vi "TelemetryMemoryUpdate.vi"   [LabVIEW 2018]
uses:
  <vilib>/rvi/Emulation/niFpgaGetClockAttributes.vi
  <vilib>/rvi/Emulation/niFpgaSctlEmulationGetInTimedLoop.vi
  <vilib>/rvi/Emulation/niFpgaEmulationReportErrorSimple.vi
  <vilib>/rvi/Emulation/niFpgaEmulationIsFPGAContextNoSignature.vi
  <vilib>/rvi/errors/niFpgaSetErrorForExecOnDevCompSimple.vi
  <vilib>/rvi/eio/common/nirviEmuReportErrorAndStop.vi
  <vilib>/rvi/DataTransferAndStorage/Container/Common/niFpgaContainerGetUniqueNameForEmu.vi
  <vilib>/rvi/FIFO/Fifo_Resource/nirvififoEmulationSetSize.vi
  <vilib>/rvi/FIFO/Fifo_Resource/nirviFifoEmulationQueueMgr.vi
  <instcachedir>/0/nirviFifoEmulationQueueMgr_E5CAEC123FF24DC58D834DCA3CDAA9B5.lvgen/nirviFifoEmulationQueueMgr_E5CAEC123FF24DC58D834DCA3CDAA9B5_022.vi
  <vilib>/Utility/error.llb/Clear Errors.vi
  <vilib>/rvi/FIFO/Fifo_Resource/nirvififoEmulationCreateLock.vi
  <vilib>/rvi/Emulation/niFpgaProcessEmulError.vi
  <vilib>/rvi/FIFO/Fifo_Resource/nirvififoEmulationObtainLock.vi
  <vilib>/rvi/FIFO/Fifo_Resource/nirvififoEmulationReleaseLock.vi
  <vilib>/rvi/occurrence/nirviWaitOnOccurrenceBase.vi
  <vilib>/rvi/errors/nirviReportUnexpectedCaseInternalError.vi
  <vilib>/rvi/errors/nirviReportUnexpectedCaseInternalError (U32).vi
  <vilib>/rvi/Emulation/niFpgaCriticalErrorInLSC.vi
  <vilib>/rvi/DataTransferAndStorage/Container/XNode/niFpgaContainer.xnode
  <vilib>/rvi/FIFO/Fifo_Resource/nirvififoEmulationRead.vi
types:
  T1 = cluster{"DataType":enum8{"U8", "U16", "U32", "U64", "I8", "I16", "I32", "I64", "SGL"}, "Mode":enum8{"=", "+", "-", "|"}, "Field":enum16{"None", "AnalogInputSampleCount", "AnalogInputSampleTimestamp", "AnalogInputRaw1", "AnalogInputRaw2", "AnalogInputRaw3", "AnalogInputRaw4", "AnalogInputRaw5", "AnalogInputRaw6", "AnalogInputRaw7", "AnalogInputRaw8", "AnalogInputRaw9", "AnalogInputRaw10", "AnalogInputRaw11", "AnalogInputRaw12", "AnalogInputRaw13", "AnalogInputRaw14", "AnalogInputRaw15", "AnalogInputRaw16", "DigitalInputSampleCount", "DigitalInputSampleTimestamp", "DigitalInputStates", "ThermocoupleSampleCount", "ThermocoupleSampleTimestamp", "ThermocoupleRaw1", "ThermocoupleRaw2", "ThermocoupleRaw3", "ThermocoupleRaw4", "ThermocoupleRaw5", "ThermocoupleRaw6", "ThermocoupleRaw7", "ThermocoupleRaw8", "ThermocoupleRaw9", "ThermocoupleRaw10", "ThermocoupleRaw11", "ThermocoupleRaw12", "ThermocoupleRaw13", "ThermocoupleRaw14", "ThermocoupleRaw15", "ThermocoupleRaw16", "WindSensorTxBytes", "WindSensorTxFrames", "WindSensorRxBytes", "WindSensorRxFrames", "WindSensorErrorTimestamp", "WindSensorErrorCode", "WindSensorSampleTimestamp", "WindSensorXRaw", "WindSensorYRaw", "WindSensorZRaw", "WindSensorSonicTempRaw", "WindSensorDiagWord", "WindSensorRecordCount", "FlowSensorTxBytes", "FlowSensorTxFrames", "FlowSensorRxBytes", "FlowSensorRxFrames", "FlowSensorErrorTimestamp", "FlowSensorErrorCode", "FlowSensorSampleTimestamp", "FlowSensorSignalStrength", "FlowSensorFlowRate", "FlowSensorNetTotalizer", "FlowSensorPositiveTotalizer", "FlowSensorNegativeTotalizer", "FlowSensorTemperature1", "FlowSensorTemperature2", "VFDTxBytes", "VFDTxFrames", "VFDRxBytes", "VFDRxFrames", "VFDErrorTimestamp", "VFDErrorCode", "VFDSampleTimestamp", "VFDVelocityBits", "VFDDiagnosticCode", "VFDFrequencyCommand", "VFDOutputFrequency", "VFDOutputCurrent", "VFDDCBusVoltage", "VFDOutputVoltage"}, "Data":u64}
  T2 = enum8{"U8", "U16", "U32", "U64", "I8", "I16", "I32", "I64", "SGL"}
  T3 = enum16{"None", "AnalogInputSampleCount", "AnalogInputSampleTimestamp", "AnalogInputRaw1", "AnalogInputRaw2", "AnalogInputRaw3", "AnalogInputRaw4", "AnalogInputRaw5", "AnalogInputRaw6", "AnalogInputRaw7", "AnalogInputRaw8", "AnalogInputRaw9", "AnalogInputRaw10", "AnalogInputRaw11", "AnalogInputRaw12", "AnalogInputRaw13", "AnalogInputRaw14", "AnalogInputRaw15", "AnalogInputRaw16", "DigitalInputSampleCount", "DigitalInputSampleTimestamp", "DigitalInputStates", "ThermocoupleSampleCount", "ThermocoupleSampleTimestamp", "ThermocoupleRaw1", "ThermocoupleRaw2", "ThermocoupleRaw3", "ThermocoupleRaw4", "ThermocoupleRaw5", "ThermocoupleRaw6", "ThermocoupleRaw7", "ThermocoupleRaw8", "ThermocoupleRaw9", "ThermocoupleRaw10", "ThermocoupleRaw11", "ThermocoupleRaw12", "ThermocoupleRaw13", "ThermocoupleRaw14", "ThermocoupleRaw15", "ThermocoupleRaw16", "WindSensorTxBytes", "WindSensorTxFrames", "WindSensorRxBytes", "WindSensorRxFrames", "WindSensorErrorTimestamp", "WindSensorErrorCode", "WindSensorSampleTimestamp", "WindSensorXRaw", "WindSensorYRaw", "WindSensorZRaw", "WindSensorSonicTempRaw", "WindSensorDiagWord", "WindSensorRecordCount", "FlowSensorTxBytes", "FlowSensorTxFrames", "FlowSensorRxBytes", "FlowSensorRxFrames", "FlowSensorErrorTimestamp", "FlowSensorErrorCode", "FlowSensorSampleTimestamp", "FlowSensorSignalStrength", "FlowSensorFlowRate", "FlowSensorNetTotalizer", "FlowSensorPositiveTotalizer", "FlowSensorNegativeTotalizer", "FlowSensorTemperature1", "FlowSensorTemperature2", "VFDTxBytes", "VFDTxFrames", "VFDRxBytes", "VFDRxFrames", "VFDErrorTimestamp", "VFDErrorCode", "VFDSampleTimestamp", "VFDVelocityBits", "VFDDiagnosticCode", "VFDFrequencyCommand", "VFDOutputFrequency", "VFDOutputCurrent", "VFDDCBusVoltage", "VFDOutputVoltage"}
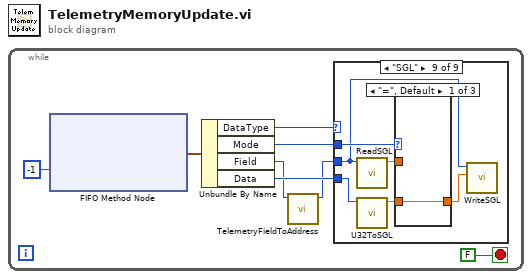
[diagram p0: block diagram]
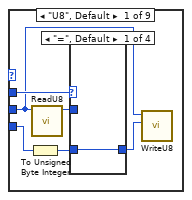
[diagram p2: hidden frame]
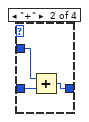
[diagram p3: hidden frame]
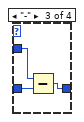
[diagram p4: hidden frame]
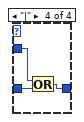
[diagram p5: hidden frame]
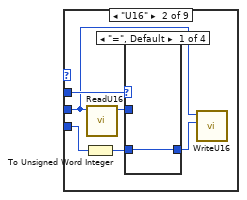
[diagram p6: hidden frame]
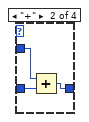
[diagram p7: hidden frame]
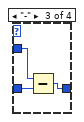
[diagram p8: hidden frame]
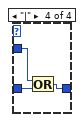
[diagram p9: hidden frame]
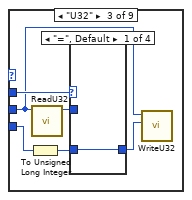
[diagram p10: hidden frame]
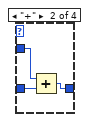
[diagram p11: hidden frame]
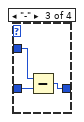
[diagram p12: hidden frame]
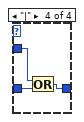
[diagram p13: hidden frame]
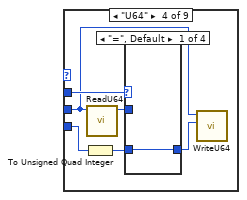
[diagram p14: hidden frame]
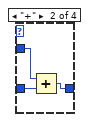
[diagram p15: hidden frame]
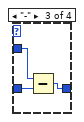
[diagram p16: hidden frame]
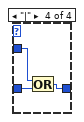
[diagram p17: hidden frame]
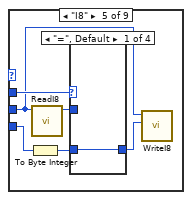
[diagram p18: hidden frame]
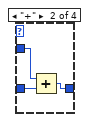
[diagram p19: hidden frame]
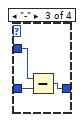
[diagram p20: hidden frame]
diagram:
  n1 = while {
    stop <- FALSE stop-if-true
    n2 = xnode ("FIFO Method Node")("Timeout"=-1) -> ("Element"=w7:T1)  [unwired: 1 in, 2 out]
    n3 = Unbundle By Name(w7) -> ("DataType"=w4:T2, "Mode"=w3:enum8{"=", "+", "-", "|"}, "Field"=w2:T3, "Data"=w6:u64)
    n4 = call "TelemetryFieldToAddress.vi"("TelemetryFields"=w2) -> ("Address"=w1:u32)  [unwired: 10 in]
    n5 = case shown="\"SGL\"" w4 {
      tunnel: w1 -> [w11 w27 w43 w59 w75 w91 w107 w123 w139]
      tunnel: w6 -> [w10 w26 w42 w58 w74 w90 w106 w122 w138]
      tunnel: w3 -> [w14 w30 w46 w62 w78 w94 w110 w126 w142]
      frame "U8", Default {
        n6 = To Unsigned Byte Integer(number=w10) -> (unsigned 8bit integer=w9:u8)
        n7 = call "ReadU8.vi"("Address"=w11) -> ("Data"=w13:u8)  [unwired: 10 in]
        n8 = case shown="\"=\", Default" w14 {
          tunnel: w9 -> [w15 w16 w19 w22]
          tunnel: [w15 w18 w21 w24] -> w12
          tunnel: w13 -> [_ w17 w20 w23]
          frame "=", Default {
          }
          frame "+" {
            n9 = Add(x=w17, y=w16) -> (x+y=w18:u8)
          }
          frame "-" {
            n10 = Subtract(x=w20, y=w19) -> (x-y=w21:u8)
          }
          frame "|" {
            n11 = Or(x=w23, y=w22) -> (x .or. y?=w24:u8)
          }
        }
        n12 = call "WriteU8.vi"("Data"=w12, "Address"=w11) -> ()  [unwired: 10 in]
      }
      frame "U16" {
        n13 = To Unsigned Word Integer(number=w26) -> (unsigned 16bit integer=w25:u16)
        n14 = call "ReadU16.vi"("Address"=w27) -> ("Data"=w29:u16)  [unwired: 10 in]
        n15 = case shown="\"=\", Default" w30 {
          tunnel: w25 -> [w31 w32 w35 w38]
          tunnel: [w31 w34 w37 w40] -> w28
          tunnel: w29 -> [_ w33 w36 w39]
          frame "=", Default {
          }
          frame "+" {
            n16 = Add(x=w33, y=w32) -> (x+y=w34:u16)
          }
          frame "-" {
            n17 = Subtract(x=w36, y=w35) -> (x-y=w37:u16)
          }
          frame "|" {
            n18 = Or(x=w39, y=w38) -> (x .or. y?=w40:u16)
          }
        }
        n19 = call "WriteU16.vi"("Data"=w28, "Address"=w27) -> ()  [unwired: 10 in]
      }
      frame "U32" {
        n20 = To Unsigned Long Integer(number=w42) -> (unsigned 32bit integer=w41:u32)
        n21 = call "ReadU32.vi"("Address"=w43) -> ("Data"=w45:u32)  [unwired: 10 in]
        n22 = case shown="\"=\", Default" w46 {
          tunnel: w41 -> [w47 w48 w51 w54]
          tunnel: [w47 w50 w53 w56] -> w44
          tunnel: w45 -> [_ w49 w52 w55]
          frame "=", Default {
          }
          frame "+" {
            n23 = Add(x=w49, y=w48) -> (x+y=w50:u32)
          }
          frame "-" {
            n24 = Subtract(x=w52, y=w51) -> (x-y=w53:u32)
          }
          frame "|" {
            n25 = Or(x=w55, y=w54) -> (x .or. y?=w56:u32)
          }
        }
        n26 = call "WriteU32.vi"("Data"=w44, "Address"=w43) -> ()  [unwired: 10 in]
      }
      frame "U64" {
        n27 = To Unsigned Quad Integer(1:w58) -> (0:w57:u64)
        n28 = call "ReadU64.vi"("Address"=w59) -> ("Data"=w61:u64)  [unwired: 10 in]
        n29 = case shown="\"=\", Default" w62 {
          tunnel: w57 -> [w63 w64 w67 w70]
          tunnel: [w63 w66 w69 w72] -> w60
          tunnel: w61 -> [_ w65 w68 w71]
          frame "=", Default {
          }
          frame "+" {
            n30 = Add(x=w65, y=w64) -> (x+y=w66:u64)
          }
          frame "-" {
            n31 = Subtract(x=w68, y=w67) -> (x-y=w69:u64)
          }
          frame "|" {
            n32 = Or(x=w71, y=w70) -> (x .or. y?=w72:u64)
          }
        }
        n33 = call "WriteU64.vi"("Data"=w60, "Address"=w59) -> ()  [unwired: 10 in]
      }
      frame "I8" {
        n34 = To Byte Integer(number=w74) -> (8bit integer=w73:i8)
        n35 = call "ReadI8.vi"("Address"=w75) -> ("Data"=w77:i8)  [unwired: 10 in]
        n36 = case shown="\"=\", Default" w78 {
          tunnel: w73 -> [w79 w80 w83 w86]
          tunnel: [w79 w82 w85 w88] -> w76
          tunnel: w77 -> [_ w81 w84 w87]
          frame "=", Default {
          }
          frame "+" {
            n37 = Add(x=w81, y=w80) -> (x+y=w82:i8)
          }
          frame "-" {
            n38 = Subtract(x=w84, y=w83) -> (x-y=w85:i8)
          }
          frame "|" {
            n39 = Or(x=w87, y=w86) -> (x .or. y?=w88:i8)
          }
        }
        n40 = call "WriteI8.vi"("Data"=w76, "Address"=w75) -> ()  [unwired: 10 in]
      }
      frame "I16" {
        n41 = To Word Integer(number=w90) -> (16bit integer=w89:i16)
        n42 = call "ReadI16.vi"("Address"=w91) -> ("Data"=w93:i16)  [unwired: 10 in]
        n43 = case shown="\"=\", Default" w94 {
          tunnel: w89 -> [w95 w96 w99 w102]
          tunnel: [w95 w98 w101 w104] -> w92
          tunnel: w93 -> [_ w97 w100 w103]
          frame "=", Default {
          }
          frame "+" {
            n44 = Add(x=w97, y=w96) -> (x+y=w98:i16)
          }
          frame "-" {
            n45 = Subtract(x=w100, y=w99) -> (x-y=w101:i16)
          }
          frame "|" {
            n46 = Or(x=w103, y=w102) -> (x .or. y?=w104:i16)
          }
        }
        n47 = call "WriteI16.vi"("Data"=w92, "Address"=w91) -> ()  [unwired: 10 in]
      }
      frame "I32" {
        n48 = To Long Integer(number=w106) -> (32bit integer=w105:i32)
        n49 = call "ReadI32.vi"("Address"=w107) -> ("Data"=w109:i32)  [unwired: 10 in]
        n50 = case shown="\"=\", Default" w110 {
          tunnel: w105 -> [w111 w112 w115 w118]
          tunnel: [w111 w114 w117 w120] -> w108
          tunnel: w109 -> [_ w113 w116 w119]
          frame "=", Default {
          }
          frame "+" {
            n51 = Add(x=w113, y=w112) -> (x+y=w114:i32)
          }
          frame "-" {
            n52 = Subtract(x=w116, y=w115) -> (x-y=w117:i32)
          }
          frame "|" {
            n53 = Or(x=w119, y=w118) -> (x .or. y?=w120:i32)
          }
        }
        n54 = call "WriteI32.vi"("Data"=w108, "Address"=w107) -> ()  [unwired: 10 in]
      }
      frame "I64" {
        n55 = To Quad Integer(1:w122) -> (0:w121:i64)
        n56 = call "ReadI64.vi"("Address"=w123) -> ("Data"=w125:i64)  [unwired: 10 in]
        n57 = case shown="\"=\", Default" w126 {
          tunnel: w121 -> [w127 w128 w131 w134]
          tunnel: [w127 w130 w133 w136] -> w124
          tunnel: w125 -> [_ w129 w132 w135]
          frame "=", Default {
          }
          frame "+" {
            n58 = Add(x=w129, y=w128) -> (x+y=w130:i64)
          }
          frame "-" {
            n59 = Subtract(x=w132, y=w131) -> (x-y=w133:i64)
          }
          frame "|" {
            n60 = Or(x=w135, y=w134) -> (x .or. y?=w136:i64)
          }
        }
        n61 = call "WriteI64.vi"("Data"=w124, "Address"=w123) -> ()  [unwired: 10 in]
      }
      frame "SGL" {
        n62 = call "ReadSGL.vi"("Address"=w139) -> ("Data"=w141:sgl)  [unwired: 10 in]
        n63 = call "U32ToSGL.vi"("U32"=w138) -> ("SGL"=w137:sgl)  [unwired: 10 in]
        n64 = case shown="\"=\", Default" w142 {
          tunnel: w137 -> [w143 w144 w147]
          tunnel: [w143 w146 w149] -> w140
          tunnel: w141 -> [_ w145 w148]
          frame "=", Default {
          }
          frame "+" {
            n65 = Add(x=w145, y=w144) -> (x+y=w146:sgl)
          }
          frame "-" {
            n66 = Subtract(x=w148, y=w147) -> (x-y=w149:sgl)
          }
        }
        n67 = call "WriteSGL.vi"("Data"=w140, "Address"=w139) -> ()  [unwired: 10 in]
      }
    }
  }
